vi "OverlayTemps.vi"(10 "Points":cluster{"X":i32, "Y":i32}[][](array[cluster]), 11 "Image":T1) -> (3 "Image Out":T1)   [LabVIEW 2022 SP3]
uses:
  <vilib>/vision/Image Controls.llb/IMAQ Image.ctl
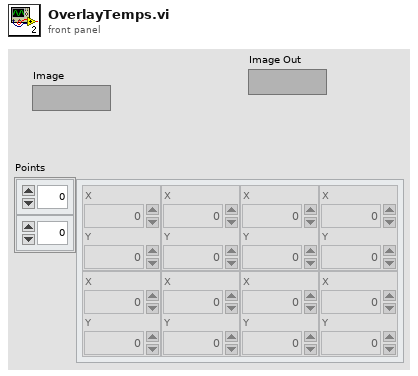
[diagram p1: front panel]
types:
  T1 = typedef "IMAQ Image.ctl" = refnum<image>
  T2 = cluster{"Desired Font (Application)":enum16{"User-specified Font", "Application Font", "System Font", "Dialog Font"}, "[User-specified Font]":cluster{"Font Name":string, "Size":i16, "Strikeout?":bool, "Italic?":bool, "Underline?":bool, "Outline?":bool, "Shadow?":bool, "Bold?":bool, "Rotation Angle":dbl}, "Horizontal Alignment":i16, "Vertical Alignment":i16}
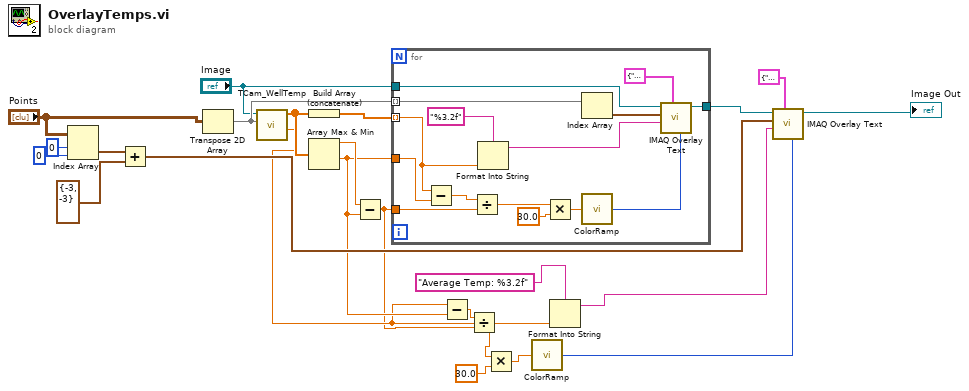
[diagram p0: block diagram]
diagram:
  n1 = Index Array(array="Points", index (row)=0, index (col)=0 ("disabled index (col)")) -> (element=w18:cluster{"X":i32, "Y":i32})
  n2 = Add(x=w18, y=cluster{"X":i32, "Y":i32} {"X"=-3, "Y"=-3}) -> (x+y=w12:cluster{"X":i32, "Y":i32})
  n3 = Transpose 2D Array(2D array="Points") -> (transposed array=w24:cluster{"X":i32, "Y":i32}[][])
  n4 = call "TCam_WellTemp.vi"("Pixels"=w24, "Image in"="Image") -> ("Mean Temp"=w9:dbl, "Temps"=w22:dbl[])  [unwired: 7 in, 1 out]
  n5 = Build Array (concatenate)(w22) -> (w20:dbl[])
  n6 = Array Max & Min(array=w22) -> (max value=w21:dbl, min value=w10:dbl)  [unwired: 2 out]
  n7 = Subtract(x=w21, y=w10) -> (x-y=w8:dbl)
  n8 = for {
    tunnel: "Image" -> [w39]
    tunnel: w24 -> [w33] mode=indexing
    tunnel: [w34] -> w13
    tunnel: w20 -> [w31] mode=indexing
    tunnel: w10 -> [w30]
    tunnel: w8 -> [w28]
    n9 = Subtract(x=w31, y=w30) -> (x-y=w29:dbl)
    n10 = Divide(x=w29, y=w28) -> (x/y=w27:dbl)
    n11 = Format Into String(format string="%3.2f", w31) -> (resulting string=w38:string)  [unwired: 2 in, 1 out]
    n12 = Multiply(x=w27, y=30.0) -> (x*y=w26:dbl)
    n13 = Index Array(array=w33) -> (element=w32:cluster{"X":i32, "Y":i32})  [unwired: 1 in]
    n14 = call "ColorRamp.vi"("Slide"=w26) -> ("Color"=w35:u32)
    n15 = call "IMAQ Overlay Text"("BG Color (Transparent)"=w35, "Font, Size & Style"=T2 {"Desired Font (Application)"=enum."Application Font", "[User-specified Font]"={"Font Name"="", "Size"=6, "Strikeout?"=FALSE, "Italic?"=FALSE, "Underline?"=FALSE, "Outline?"=FALSE, "Shadow?"=FALSE, "Bold?"=FALSE, "Rotation Angle"=0.0}, "Horizontal Alignment"=0, "Vertical Alignment"=1}, "String"=w38, "Origin"=w32, "Image"=w39) -> ("Image Out"=w34:T1)  [unwired: 5 in, 1 out]
  }
  n16 = Subtract(x=w9, y=w10) -> (x-y=w7:dbl)
  n17 = Divide(x=w7, y=w8) -> (x/y=w6:dbl)
  n18 = Multiply(x=w6, y=30.0) -> (x*y=w4:dbl)
  n19 = call "ColorRamp.vi"("Slide"=w4) -> ("Color"=w3:u32)
  n20 = Format Into String(format string="Average Temp: %3.2f", w9) -> (resulting string=w2:string)  [unwired: 2 in, 1 out]
  n21 = call "IMAQ Overlay Text"("BG Color (Transparent)"=w3, "Font, Size & Style"=T2 {"Desired Font (Application)"=enum."Application Font", "[User-specified Font]"={"Font Name"="", "Size"=6, "Strikeout?"=FALSE, "Italic?"=FALSE, "Underline?"=FALSE, "Outline?"=FALSE, "Shadow?"=FALSE, "Bold?"=FALSE, "Rotation Angle"=0.0}, "Horizontal Alignment"=0, "Vertical Alignment"=1}, "String"=w2, "Origin"=w12, "Image"=w13) -> ("Image Out"=→"Image Out":T1)  [unwired: 5 in, 1 out]
